vi "AMZ_S3_APIHLP_Parse Setup Bucket Notification Response.vi"(8 "error in (no error)":errorcluster, 11 "Response header":string) -> (0 "error out":errorcluster, 3 "Test message id":string)   [LabVIEW 2015, in "LV Interface for Amazon S3.lvlib"]
uses:
  LV Interface for Amazon S3.lvlib
  <vilib>/regexp/Match Regular Expression.xnode
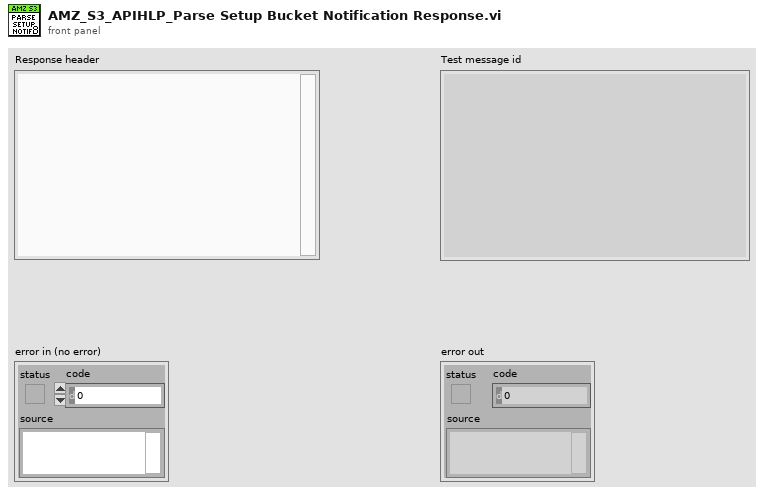
[diagram p1: front panel]
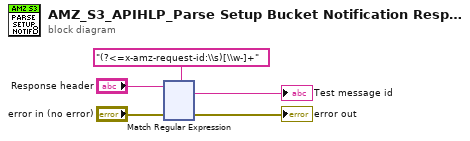
[diagram p0: block diagram]
diagram:
  n1 = xnode "Match Regular Expression"("input string"="Response header", "regular expression"="(?<=x-amz-request-id:\\s)[\\w-]+", "error in"="error in (no error)") -> ("whole match"=→"Test message id":string, "error out"=→"error out":errorcluster)  [unwired: 3 in, 3 out]
